vi "StartStopGen.vi"(10 "AOLZ":dbl=0.0001 format="%#_13g", 11 "X-Y-Z coordinates":T2 {"ROI group ID" format="%#_6f"; "Laser Power (%)" format="%#_6f"; "Zoom" format="%#_6f"; "Frame Size" format="%#_6f"; "Number of lines" format="%#_6f"; "Composite ID" format="%#_6f"; "Angle (deg)" format="%#_6f"; "ROI Time (ns)" format="%#_6f"; "ROI ID" format="%#_6f"; "Pixels in ROI" format="%#_6f"; "ROI index" format="%#_6f"; "Z stop" format="%#_6f"; "Y stop" format="%#_6f"; "X stop" format="%#_6f"; "Z start" format="%#_6f"; "X start" format="%#_6f"; "Y start" format="%#_6f"}) -> (3 "ROI Coordinates (broken down to miniscans)":T1)   [LabVIEW 2013]
uses:
  User Interface/Visualisation/Functional Imaging Viewer/Typedefs/ROI parameters data type.ctl
  Typedefs/ROI XY coordinates cluster.ctl
  Global Variables/gl_UI Ctrl Refs.vi
panel:
  out "Yc":dbl format="%#_13g"
  out "Xc":dbl format="%#_13g"
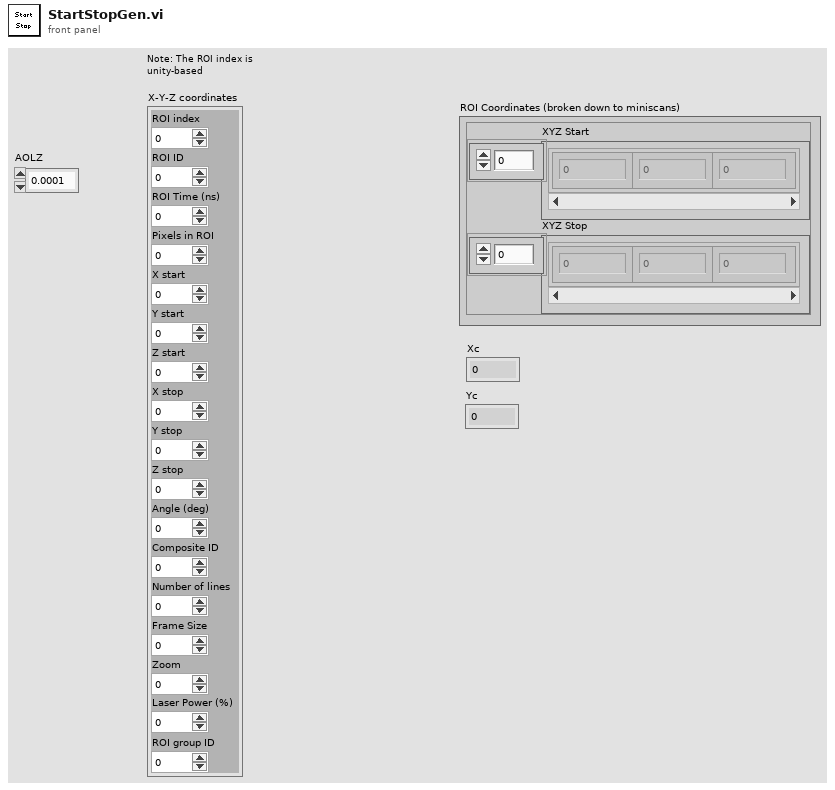
[diagram p1: front panel]
types:
  T1 = typedef "ROI XY coordinates cluster.ctl" = cluster{"XYZ Start":cluster{"X":sgl, "Y":sgl, "Z":sgl}[], "XYZ Stop":cluster{"X":sgl, "Y":sgl, "Z":sgl}[]}
  T2 = typedef "ROI parameters data type.ctl" = cluster{"ROI index":dbl, "ROI ID":dbl, "ROI Time (ns)":dbl, "Pixels in ROI":dbl, "X start":dbl, "Y start":dbl, "Z start":dbl, "X stop":dbl, "Y stop":dbl, "Z stop":dbl, "Angle (deg)":dbl, "Composite ID":dbl, "Number of lines":dbl, "Frame Size":dbl, "Zoom":dbl, "Laser Power (%)":dbl, "ROI group ID":dbl}
  T3 = typedef "UI ctrl refs cluster.ctl" = cluster{"Top level VI path":path, "Top level VI ref":refnum<vi>, "User menu ref":refnum<k9>, "Sub Panel control":refnum<vi>, "Imaging Param Tab":refnum<vi>, "Occurrence-Start drivers":refnum<k4>, "Occurrence-Speed logging initialised":refnum<k4>, "Occurrence-XYZ stage initialised":refnum<k4>, "Exit button":refnum<vi>, "Status ind":refnum<vi>, "Return to Origin":refnum<vi>, "Speed Logging":refnum<vi>, "Time Lapse":refnum<vi>, "Live Imaging":refnum<vi>, "AOL Z Stack":refnum<vi>, "Motor Z Stack":refnum<vi>, "Funct Acq button":refnum<vi>, "Hard Shutter":refnum<vi>, "Virtual Shutter":refnum<vi>, "Laser Power":refnum<vi>, "AOL Mode":refnum<vi>, "Frame Size":refnum<vi>, "Field of View":refnum<vi>, "Dwell Time":refnum<vi>, "Zoom":refnum<vi>, "AOL Z":refnum<vi>, "Objective":refnum<vi>, "Axis":refnum<vi>, "Paths & Names":refnum<vi>, "Experiment folder path (ind.)":refnum<vi>, "Last State (Ind.)":refnum<vi>, "Laser wavelength ind (nm)":refnum<vi>, "Averages":refnum<vi>, "Angle (degrees)":refnum<vi>, "X centre":refnum<vi>, "Y centre":refnum<vi>, "Plane Mode":refnum<vi>, "# Planes":refnum<vi>, "Z Start":refnum<vi>, "Z Stop":refnum<vi>, "Z Step":refnum<vi>, "PMT 1":refnum<vi>, "PMT 2":refnum<vi>, "Stage XYZ Position":refnum<vi>, "Pockels@Z Start":refnum<vi>, "Pockels@Z Stop":refnum<vi>, "Obtain Z Start":refnum<vi>, "Obtain Z Stop":refnum<vi>, "Live stim.trig.period":refnum<vi>, "Live stim.trig.enable":refnum<vi>, "Funct. Acq. Pockels Modulation":refnum<vi>, "Enable Video Recording":refnum<vi>, "Video Record-Live Imaging":refnum<vi>, "Video Record-Funct acq":refnum<vi>, "AOL Z-stack Chirps Ready (ind)":refnum<vi>, "Center freq ind (nm)":refnum<vi>, "Logging queue (ind)":refnum<vi>, "Back aperture power (ind.)":refnum<vi>, "Power after objective (ind.)":refnum<vi>, "Switch user":refnum<vi>}
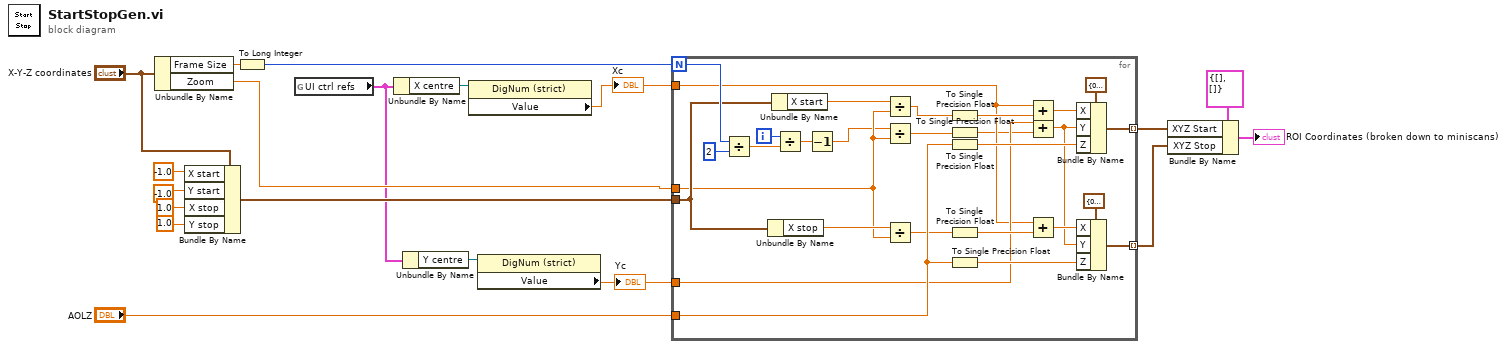
[diagram p0: block diagram]
diagram:
  n1 = Unbundle By Name("X-Y-Z coordinates") -> ("Frame Size"=w15:dbl, "Zoom"=w6:dbl)
  n2 = Bundle By Name(cluster="X-Y-Z coordinates", "X start"=-1.0, "Y start"=-1.0 ("X start"), "X stop"=1.0, "Y stop"=1.0 ("X stop")) -> (w7:T2)
  n3 = To Long Integer(number=w15) -> (32bit integer=w18:i32)
  n4 = global read "gl_UI Ctrl Refs.vi" "UI ctrl refs"() -> (w1:T3)
  n5 = Unbundle By Name(w1) -> ("X centre"=w5:refnum<vi>)
  n6 = Unbundle By Name(w1) -> ("Y centre"=w3:refnum<vi>)
  n7 = property class="DigNum (strict)"(reference=w5) -> ("Value"=w4:dbl)  [unwired: 1 in, 2 out]
  "Xc" <- w4
  n8 = property class="DigNum (strict)"(reference=w3) -> ("Value"=w2:dbl)  [unwired: 1 in, 2 out]
  "Yc" <- w2
  n9 = for {
    N: w18 -> [w47]
    tunnel: "AOLZ" -> [w40]
    tunnel: w7 -> [w36]
    tunnel: [w38] -> w17 mode=indexing
    tunnel: [w37] -> w16 mode=indexing
    tunnel: w2 -> [w31]
    tunnel: w4 -> [w30]
    tunnel: w6 -> [w24]
    i -> [w44]
    n10 = Divide(x=w47, y=2) -> (x/y=w45:dbl)
    n11 = Unbundle By Name(w36) -> ("X stop"=w26:dbl)
    n12 = Unbundle By Name(w36) -> ("X start"=w29:dbl)
    n13 = Divide(x=w44, y=w45) -> (x/y=w21:dbl)
    n14 = Decrement(x=w21) -> (x-1=w20:dbl)
    n15 = Divide(x=w29, y=w24) -> (x/y=w28:dbl)
    n16 = Divide(x=w20, y=w24) -> (x/y=w27:dbl)
    n17 = Divide(x=w26, y=w24) -> (x/y=w25:dbl)
    n18 = To Single Precision Float(number=w28) -> (single precision float=w34:sgl)
    n19 = To Single Precision Float(number=w27) -> (single precision float=w23:sgl)
    n20 = To Single Precision Float(number=w40) -> (single precision float=w42:sgl)
    n21 = To Single Precision Float(number=w25) -> (single precision float=w33:sgl)
    n22 = To Single Precision Float(number=w40) -> (single precision float=w41:sgl)
    n23 = Add(x=w30, y=w34) -> (x+y=w35:dbl)
    n24 = Add(x=w31, y=w23) -> (x+y=w22:dbl)
    n25 = Add(x=w30, y=w33) -> (x+y=w32:dbl)
    n26 = Bundle By Name(cluster=cluster{"X":sgl, "Y":sgl, "Z":sgl} {"X"=0.0, "Y"=0.0, "Z"=0.0} ("XYZ"), "X"=w35, "Y"=w22, "Z"=w42) -> (w37:cluster{"X":sgl, "Y":sgl, "Z":sgl})
    n27 = Bundle By Name(cluster=cluster{"X":sgl, "Y":sgl, "Z":sgl} {"X"=0.0, "Y"=0.0, "Z"=0.0} ("XYZ"), "X"=w32, "Y"=w22, "Z"=w41) -> (w38:cluster{"X":sgl, "Y":sgl, "Z":sgl})
  }
  n28 = Bundle By Name(cluster=T1 {"XYZ Start"=[], "XYZ Stop"=[]} ("ROI Coordinates (broken down to miniscans)"), "XYZ Start"=w16, "XYZ Stop"=w17) -> (→"ROI Coordinates (broken down to miniscans)":T1)
